vi "Build Check High Priority Time.vi"(6 "Group":i32, 7 "Virtual Memory Unit in":refnum<class "Virtual Memory Unit.lvclass">, 8 "error in (no error)":errorcluster, 10 "Starting Address":u16 format="%04x", 11 "Major Frame in":refnum<class "Major Frame.lvclass">) -> (0 "error out":errorcluster, 2 "Next Available Address":u16 format="%04x", 3 "Major Frame out":refnum<class "Major Frame.lvclass">, 5 "Virtual Memory Unit out":refnum<class "Virtual Memory Unit.lvclass">)   [LabVIEW 2016, in "BCI-1553 API.lvlib" / "Major Frame.lvclass"]
doc: "Checks if there's enough time to run a high-priority async message."
uses:
  Major Frame.lvclass
  Dependencies/Virtual Memory Unit/Virtual Memory Unit.lvclass
  BCI-1553 API.lvlib
  TypeDefs/BC Condition Codes.ctl
  TypeDefs/BC Op Codes - Verbose.ctl
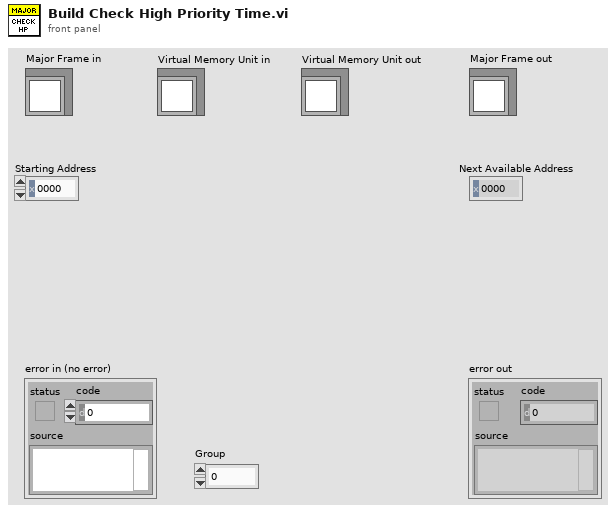
[diagram p1: front panel]
types:
  T1 = typedef "BCI-1553 API.lvlib/BC Op Codes - Verbose.ctl" = enum16{"EXECUTE MSG", "EXECUTE MSG GO", "JUMP", "CALL SUBROUTINE", "RETURN", "INTERRUPT REQUEST", "HALT", "DELAY", "WAIT FRAME TIMER = 0", "COMPARE FRAME TIMER", "COMPARE MSG TIMER", "LOAD TIME TAG CTR", "LOAD TIME TAG CTR HI", "LOAD FRAME TIMER", "START FRAME TIMER", "PUSH TIME TAG COUNT", "PUSH TIME TAG COUNT HI", "PUSH TIME TAG COUNT BOTH", "PUSH BLOCK STATUS WORD", "PUSH CURRENT VALUE", "PUSH INDIRECT", "WAIT EXT TRIGGER", "EXECUTE AND FLIP", "EXECUTE, FLIP, GO", "WRITE VALUE TO WMI", "WRITE VALUE TO MEM", "DECREMENT RAM, SKIP", "FLAG"}
  T2 = typedef "BCI-1553 API.lvlib/BC Condition Codes.ctl" = enum16{"GP0 == 1 || LT", "GP1 == 1 || NE", "GP2 == 1", "GP3 == 1", "GP4 == 1", "GP5 == 1", "GP6 == 1", "GP7 == 1", "NORESP", "FMTERR", "GOODBLOCK", "MSKSTATSET", "BADMSG", "1RETRY", "2RETRY", "ALWAYS"}
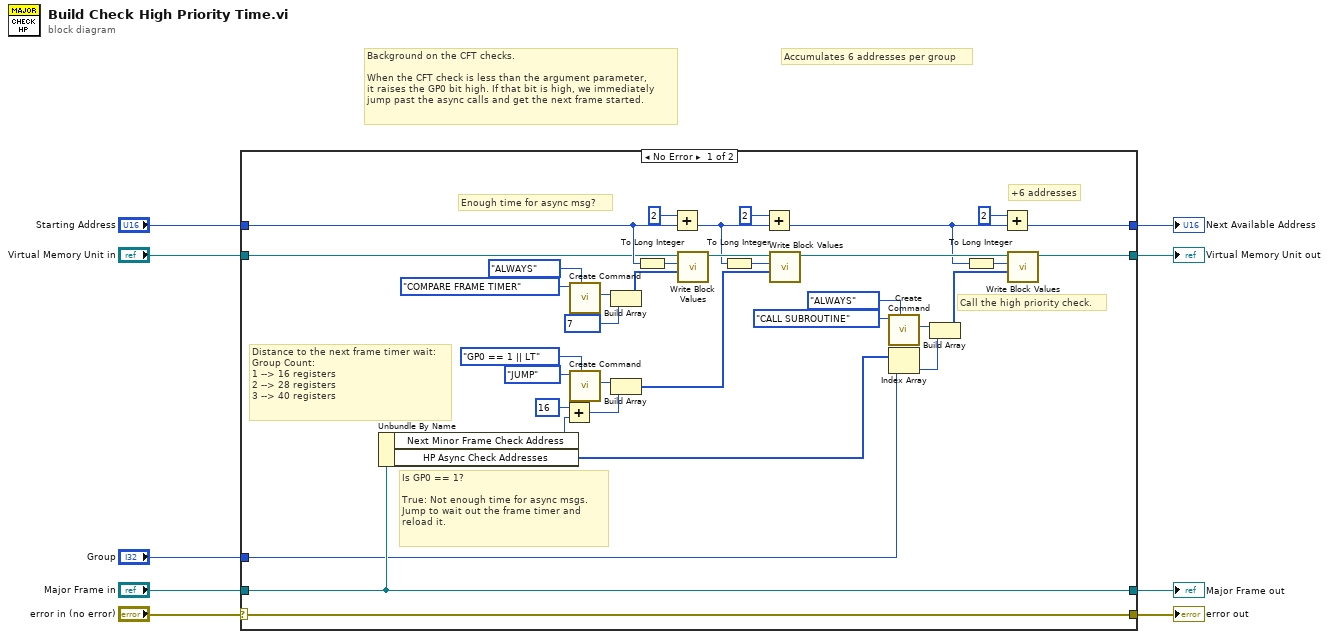
[diagram p0: block diagram]
diagram:
  # "Background on the CFT checks.\n\nWhen the CFT check is less than the argument parameter,\nit raises the GP0 bit high. If that bit is high, we immediately\njump past the async calls and get the next frame started."
  # "Accumulates 6 addresses per group"
  n1 = case shown="No Error" "error in (no error)" {
    selector: "error in (no error)" -> [w44 w48]
    tunnel: [w44 w48] -> w8
    tunnel: [w14 w47] -> w6
    tunnel: "Major Frame in" -> [w14 w47]
    tunnel: "Group" -> [w13 _]
    tunnel: "Starting Address" -> [w26 w46]
    tunnel: "Virtual Memory Unit in" -> [w25 w45]
    tunnel: [w12 w45] -> w2
    tunnel: [w11 w46] -> w1
    frame No Error {
      # "+6 addresses"
      # "Is GP0 == 1?\n\nTrue: Not enough time for async msgs.\nJump to wait out the frame timer and\nreload it."
      # "Call the high priority check."
      # "Distance to the next frame timer wait:\nGroup Count:\n1 --> 16 registers\n2 --> 28 registers\n3 --> 40 registers"
      # "Enough time for async msg?"
      n2 = Unbundle By Name(w14) -> ("Next Minor Frame Check Address"=w17:u16, "HP Async Check Addresses"=w10:u16[])
      n3 = Add(x=u16 16 ("element"), y=w17) -> (x+y=w28:u16)
      n4 = call "Create Command.vi"("Condition"=BC_Condition_Codes."ALWAYS", "Op Code"=BC_Op_Codes_-_Verbose."COMPARE FRAME TIMER") -> ("Instruction"=w41:u16)  [unwired: 8 in, 1 out]
      n5 = call "Create Command.vi"("Condition"=BC_Condition_Codes."GP0 == 1 || LT", "Op Code"=BC_Op_Codes_-_Verbose."JUMP") -> ("Instruction"=w35:u16)  [unwired: 8 in, 1 out]
      n6 = Build Array(w41, u16 7 ("element")) -> (w39:u16[])
      n7 = Build Array(w35, w28) -> (w36:u16[])
      n8 = To Long Integer(number=w26) -> (32bit integer=w38:i32)
      n9 = Add(x=u16 2, y=w26) -> (x+y=w31:u16)
      n10 = call "Write Block Values.vi"("Write Block"=w39, "Start Index"=w38, "Virtual Memory Unit in"=w25) -> ("Virtual Memory Unit out"=w32:refnum<class "Virtual Memory Unit.lvclass">)  [unwired: 7 in, 1 out]
      n11 = To Long Integer(number=w31) -> (32bit integer=w37:i32)
      n12 = Add(x=u16 2, y=w31) -> (x+y=w15:u16)
      n13 = call "Write Block Values.vi"("Write Block"=w36, "Start Index"=w37, "Virtual Memory Unit in"=w32) -> ("Virtual Memory Unit out"=w16:refnum<class "Virtual Memory Unit.lvclass">)  [unwired: 7 in, 1 out]
      n14 = call "Create Command.vi"("Condition"=BC_Condition_Codes."ALWAYS", "Op Code"=BC_Op_Codes_-_Verbose."CALL SUBROUTINE") -> ("Instruction"=w21:u16)  [unwired: 8 in, 1 out]
      n15 = Index Array(array=w10, index=w13) -> (element=w23:u16)
      n16 = Build Array(w21, w23) -> (w22:u16[])
      n17 = To Long Integer(number=w15) -> (32bit integer=w18:i32)
      n18 = Add(x=u16 2, y=w15) -> (x+y=w11:u16)
      n19 = call "Write Block Values.vi"("Write Block"=w22, "Start Index"=w18, "Virtual Memory Unit in"=w16) -> ("Virtual Memory Unit out"=w12:refnum<class "Virtual Memory Unit.lvclass">)  [unwired: 7 in, 1 out]
    }
    frame Error {
    }
  }
  "error out" <- w8
  "Major Frame out" <- w6
  "Virtual Memory Unit out" <- w2
  "Next Available Address" <- w1
